vi "Graphics_GetClassAttributes.vi"(0 "reference in":refnum<class "Graphics.lvclass">, 5 "error in (no error)":errorcluster) -> (14 "reference out":refnum<class "Graphics.lvclass">, 16 "Class attributes":T1, 17 "Attributes locked?":bool, 19 "error out":errorcluster)   [LabVIEW 2012, in "Graphics.lvclass"]
doc: "Returns the class attributes of a Graphics or a sub class. If reference is wired, the class attributes of the class (or sub class) will be returned else the class attributes will default to the Graphics class.\n\nIf the data is currently locked for modification, 'Attributes locked?' will return TRUE. If reference is wired, the class attributes of the class (or sub class) will be returned else the class attributes of the Graphics.\n\n[GOOP 2.0.15]"
uses:
  <resource>/Framework/Providers/Open_GDS/UML/Graphics_class/Graphics.lvclass
  <resource>/Framework/Providers/Open_GDS/UML/Graphics_class/protected/ClassAttributes.ctl
  <vilib>/addons/_goop3.llb/3GOOPStates.ctl
  <resource>/Framework/Providers/Open_GDS/UML/Graphics_class/Graphics.lvclass/Graphics.ctl
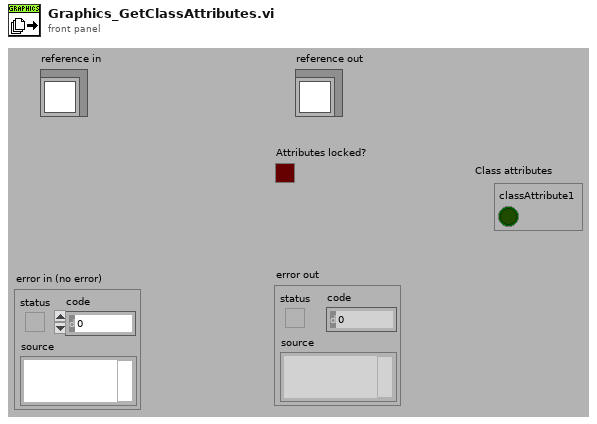
[diagram p1: front panel]
types:
  T1 = typedef "Graphics.lvclass/ClassAttributes.ctl" = cluster{"classAttribute1":bool}
  T2 = typedef "3GOOPStates.ctl" = enum16{"Set", "Get", "New", "Delete", "Clear", "Test and get", "Unlock data", "Information", "Look up existing", "New or look up existing", "Test and get shared", "Get shared", "Set shared", "Unlock shared", "Find dynamic method", "Register dynamic method", "Preload dynamic method", "Probe", "Cast to more generic", "Cast to more specific"}
  T3 = typedef "Graphics.lvclass/ObjectReference.ctl" = refnum<k1>
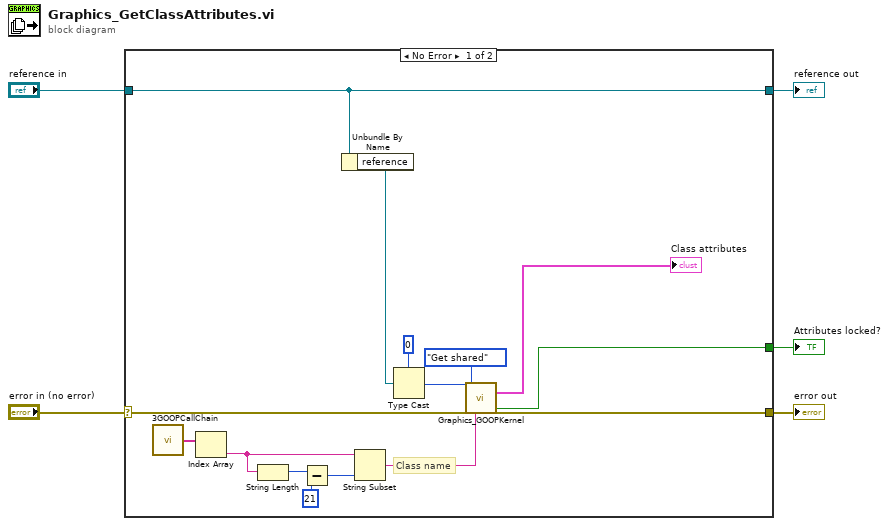
[diagram p0: block diagram]
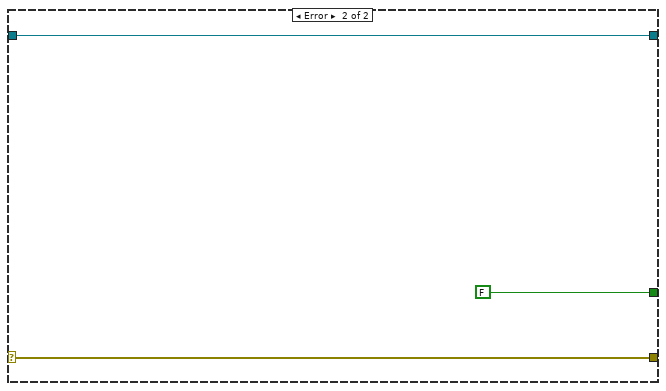
[diagram p2: hidden frame]
diagram:
  n1 = case shown="No Error" "error in (no error)" {
    selector: "error in (no error)" -> [w15 w22]
    tunnel: [w17 w23] -> w5
    tunnel: [w20 w22] -> w4
    tunnel: "reference in" -> [w17 w23]
    tunnel: [w19 FALSE ("Data locked?")] -> w1
    frame No Error {
      # "Class name"
      n2 = call <vilib>:"3GOOPCallChain.vi"() -> ("call chain"=w10:string[])
      n3 = Index Array(array=w10) -> (element=w7:string)  [unwired: 1 in]
      n4 = String Length(string=w7) -> (length=w12:i32)
      n5 = Subtract(x=w12, y=21) -> (x-y=w9:i32)
      n6 = Unbundle By Name(w17) -> ("reference"=w6:T3)
      n7 = String Subset(string=w7, length (rest)=w9) -> (substring=w8:string)  [unwired: 1 out]
      n8 = Type Cast(type=0, x=w6) -> (*(type *) &x=w18:i32)
      n9 = call <resource>:"Graphics_GOOPKernel.vi"("Ref in"=w18, "error in (no error)"=w15, "Action"=3GOOPStates."Get shared", "Dynamic VI name"=w8) -> ("Data shared out"=→"Class attributes":T1, "Data locked?"=w19:bool, "error out"=w20:errorcluster)  [unwired: 11 in, 10 out]
    }
    frame Error {
    }
  }
  "error out" <- w4
  "reference out" <- w5
  "Attributes locked?" <- w1
